vi "Check Score.vi"(8 "error in (no error)":errorcluster, 10 "End":bool, 11 "Board_Game in":refnum<class "Board_Game.lvclass">) -> (0 "error out":errorcluster, 3 "Board_Game out":refnum<class "Board_Game.lvclass">)   [LabVIEW 2021, in "Board_Game.lvclass"]
uses:
  Board_Game.lvclass
  Board_Game.lvclass/Board_Game.ctl
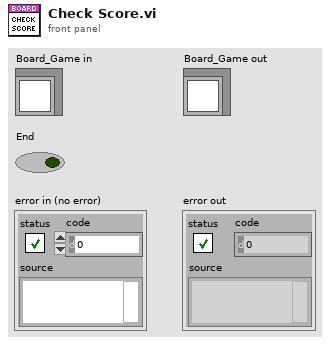
[diagram p1: front panel]
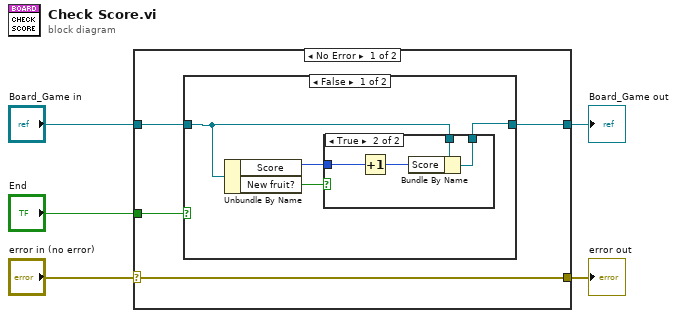
[diagram p0: block diagram]
diagram:
  n1 = case shown="No Error" "error in (no error)" {
    selector: "error in (no error)" -> [w9 w21]
    tunnel: [w9 w21] -> w4
    tunnel: [w6 w20] -> w2
    tunnel: "Board_Game in" -> [w7 w20]
    tunnel: "End" -> [w8 _]
    frame No Error {
      n2 = case shown="False" w8 {
        tunnel: w7 -> [w13 w19]
        tunnel: [w12 w19] -> w6
        frame False {
          n3 = Unbundle By Name(w13) -> ("Score"=w11:u32, "New fruit?"=w10:bool)
          n4 = case shown="True" w10 {
            tunnel: w13 -> [w14 w18]
            tunnel: [w14 w17] -> w12
            tunnel: w11 -> [_ w16]
            frame False {
            }
            frame True {
              n5 = Increment(x=w16) -> (x+1=w15:u32)
              n6 = Bundle By Name(cluster=w18, "Score"=w15) -> (w17:refnum<class "Board_Game.lvclass">)
            }
          }
        }
        frame True {
        }
      }
    }
    frame Error {
    }
  }
  "error out" <- w4
  "Board_Game out" <- w2
